vi "ControlNameUnescape.vi"(11 "escaped string":string) -> (3 "label":string)   [LabVIEW 2019, in "SetGetControlValue.lvlib"]
uses:
  SetGetControlValue.lvlib
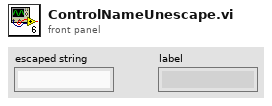
[diagram p1: front panel]
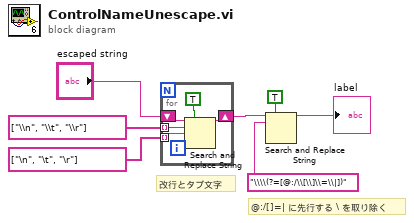
[diagram p0: block diagram]
diagram:
  # "改行とタブ文字"
  # "@:/[]=| に先行する \\ を取り除く"
  n1 = for {
    tunnel: string[] ["\\n", "\\t", "\\r"] ("search string") -> [w12] mode=indexing
    tunnel: string[] ["\n", "\t", "\r"] ("search string") -> [w11] mode=indexing
    shift-right: [w9] -> w1
    shift-left: "escaped string" -> [w10]
    n2 = Search and Replace String(replace all?=TRUE ("replace all? (F)"), input string=w10, search string=w12, replace string=w11) -> (result string=w9:string)  [unwired: 4 in, 3 out]
  }
  n3 = Search and Replace String(replace all?=TRUE ("replace all? (F)"), input string=w1, search string="\\\\(?=[@:/\\[\\]\\=\\|])") -> (result string=→"label":string)  [unwired: 5 in, 3 out]
